vi "tatrocki_host_C.vi"() -> ()   [LabVIEW 2020]
panel:
  in  "SignalSend":bool
  in  "Stop":bool
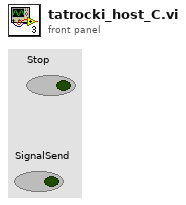
[diagram p1: front panel]
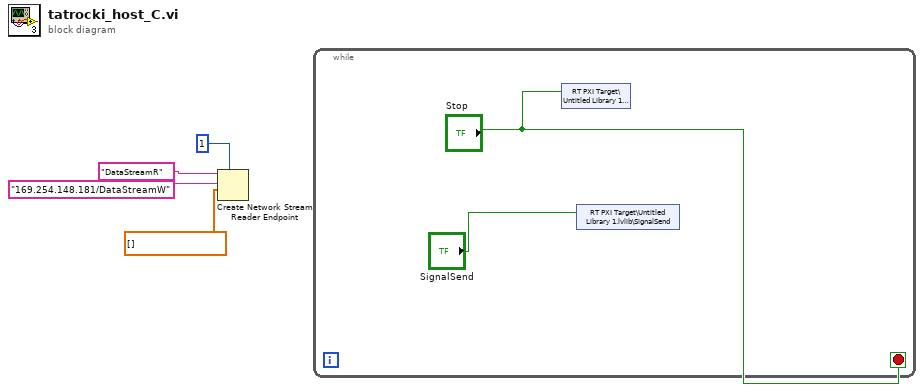
[diagram p0: block diagram]
diagram:
  n1 = Create Network Stream Reader Endpoint(7:1 ("reader buffer size"), 9:dbl[] [], 10:"169.254.148.181/DataStreamW" ("writer url"), 11:"DataStreamR" ("reader name")) -> ()  [unwired: 3 in, 2 out]
  n2 = while {
    stop <- "Stop" stop-if-true
    n3 = shared-variable "RT PXI Target\\Untitled Library 1.lvlib\\Stop"("Stop") -> ()  [unwired: 1 in, 1 out]
    n4 = shared-variable "RT PXI Target\\Untitled Library 1.lvlib\\SignalSend"("SignalSend") -> ()  [unwired: 1 in, 1 out]
  }
